vi "Front_measurement.vi"(8 "error in":errorcluster, 10 "AI duration (ms)":i32=1000, 11 "Digital Ports":tag="Dev1/port0") -> (1 "error out":errorcluster, 2 "data":waveform(dbl))   [LabVIEW 2021]
uses:
  <vilib>/DAQmx/write.llb/DAQmx Write (Digital 1D U32 1Chan NSamp).vi
  <vilib>/DAQmx/read.llb/DAQmx Read (Analog Wfm 1Chan NSamp).vi
  <vilib>/DAQmx/create/channels.llb/DAQmx Create Channel (DO-Digital Output).vi
  <vilib>/DAQmx/create/channels.llb/DAQmx Create Channel (CO-Pulse Generation-Ticks).vi
  <vilib>/DAQmx/configure/timing.llb/DAQmx Timing (Implicit).vi
  <vilib>/DAQmx/create/channels.llb/DAQmx Create Channel (AI-Voltage-Basic).vi
  <vilib>/DAQmx/configure/timing.llb/DAQmx Timing (Sample Clock).vi
  <vilib>/DAQmx/configure/trigger.llb/DAQmx Start Trigger (Analog Edge).vi
  Addons/DAQ_Pulse_Gen/Global_DAQ.vi
  <vilib>/DAQmx/miscellaneous.llb/DAQmx Fill In Error Info.vi
  <vilib>/DAQmx/create/channels.llb/DAQmx Create Channel (CO-Pulse Generation-Frequency).vi
  <vilib>/Utility/error.llb/Error Cluster From Error Code.vi
  <vilib>/ErrorRing/Error Ring.xnode
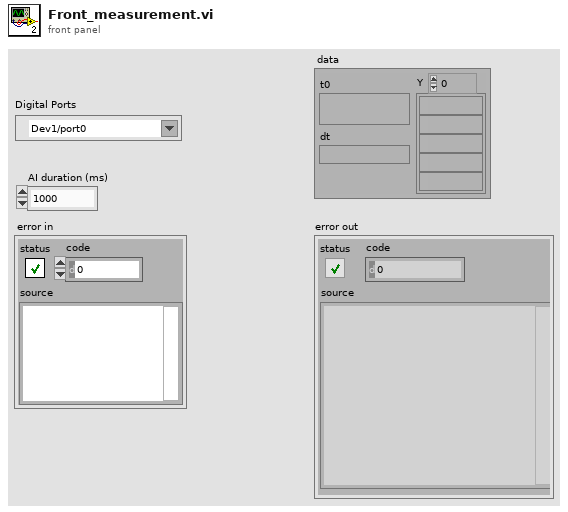
[diagram p1: front panel]
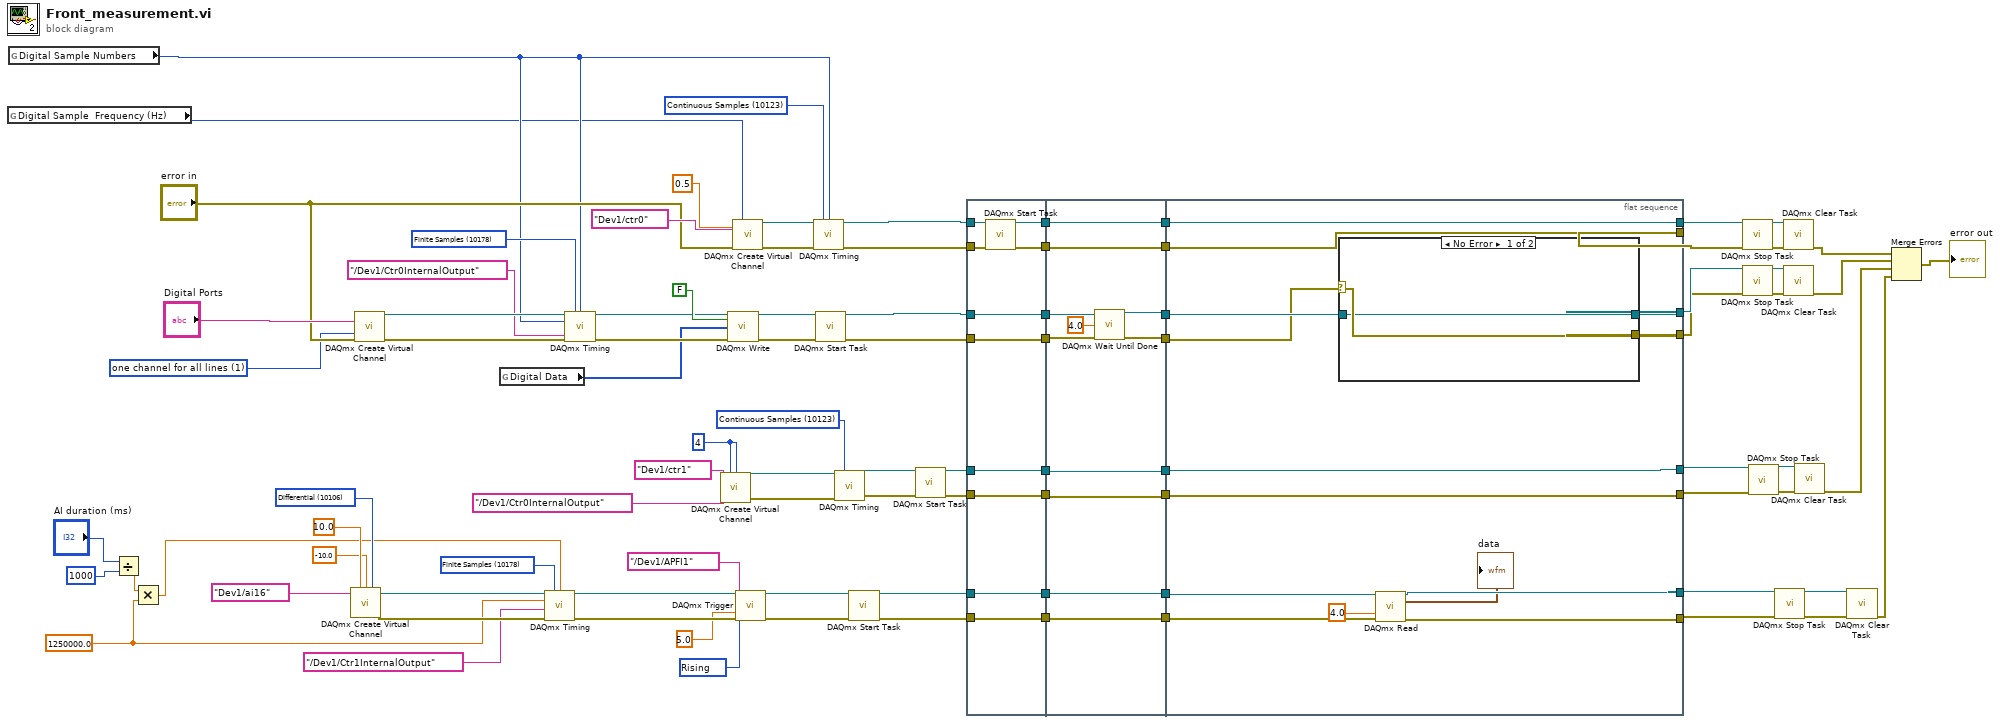
[diagram p0: block diagram]
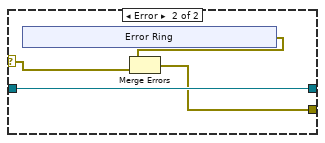
[diagram p2: hidden frame]
diagram:
  w3 = 1250000.0 ("rate")
  w26 = 10106 items=["Default"=-1, "RSE"=10083, "NRSE"=10078, "Differential"=10106, "Pseudodifferential"=12529] ("input terminal configuration")
  w28 = 10280 items=["Rising"=10280, "Falling"=10171] ("slope")
  w37 = 10178 items=["Finite Samples"=10178, "Continuous Samples"=10123, "Hardware Timed Single Point"=12522] ("sample mode")
  w55 = 10123 items=["Finite Samples"=10178, "Continuous Samples"=10123, "Hardware Timed Single Point"=12522] ("sample mode")
  w56 = u32 4 ("low ticks")
  w76 = 1 items=["one channel for each line", "one channel for all lines"] ("line grouping")
  w78 = 10123 items=["Finite Samples"=10178, "Continuous Samples"=10123, "Hardware Timed Single Point"=12522] ("sample mode")
  w86 = 10178 items=["Finite Samples"=10178, "Continuous Samples"=10123, "Hardware Timed Single Point"=12522] ("sample mode")
  n1 = global read "Global_DAQ.vi" "Digital Sample  Frequency (Hz)"() -> (w6:u32)
  n2 = global read "Global_DAQ.vi" "Digital Sample Numbers"() -> (w9:u32)
  n3 = Divide(x="AI duration (ms)", y=1000) -> (x/y=w4:dbl)
  n4 = Multiply(x=w4, y=w3) -> (x*y=w1:dbl)
  n5 = call-poly <vilib>:"DAQmx Create Virtual Channel.vi"("maximum value"=10.0, "minimum value"=-10.0, "input terminal configuration"=w26, "physical channels"=tag "Dev1/ai16") -> ("task out"=w47:refnum<k21>, "error out"=w46:errorcluster)  [unwired: 10 in]
  n6 = call-poly <vilib>:"DAQmx Create Virtual Channel.vi"("lines"="Digital Ports", "line grouping"=w76, "error in"="error in") -> ("task out"=w89:refnum<k21>, "error out"=w88:errorcluster)  [unwired: 11 in]
  n7 = global read "Global_DAQ.vi" "Digital Data"() -> (w77:u32[])
  n8 = call-poly <vilib>:"DAQmx Timing.vi"("task/channels in"=w47, "sample mode"=w37, "samples per channel"=w1, "rate"=w3, "source"=tag "/Dev1/Ctr1InternalOutput", "error in"=w46) -> ("task out"=w44:refnum<k21>, "error out"=w43:errorcluster)  [unwired: 8 in]
  n9 = call-poly <vilib>:"DAQmx Timing.vi"("task/channels in"=w89, "sample mode"=w86, "samples per channel"=w9, "rate"=w9, "source"=tag "/Dev1/Ctr0InternalOutput", "error in"=w88) -> ("task out"=w80:refnum<k21>, "error out"=w79:errorcluster)  [unwired: 8 in]
  n10 = call-poly <vilib>:"DAQmx Create Virtual Channel.vi"("high ticks"=w56, "low ticks"=w56, "counter"=tag "Dev1/ctr1", "source of ticks"=tag "/Dev1/Ctr0InternalOutput") -> ("task out"=w58:refnum<k21>, "error out"=w57:errorcluster)  [unwired: 10 in]
  n11 = call-poly <vilib>:"DAQmx Write.vi"("task/channels in"=w80, "auto start"=FALSE, "data"=w77, "error in"=w79) -> ("task out"=w83:refnum<k21>, "error out"=w82:errorcluster)  [unwired: 9 in, 1 out]
  n12 = call-poly <vilib>:"DAQmx Create Virtual Channel.vi"("frequency"=w6, "duty cycle"=0.5, "counter"=tag "Dev1/ctr0", "error in"="error in") -> ("task out"=w84:refnum<k21>, "error out"=w90:errorcluster)  [unwired: 10 in]
  n13 = call-poly <vilib>:"DAQmx Trigger.vi"("task/channels in"=w44, "source"=tag "/Dev1/APFI1", "slope"=w28, "level"=5.0, "error in"=w43) -> ("task out"=w41:refnum<k21>, "error out"=w40:errorcluster)  [unwired: 9 in]
  n14 = call-poly <vilib>:"DAQmx Timing.vi"("task/channels in"=w84, "sample mode"=w78, "samples per channel"=w9, "error in"=w90) -> ("task out"=w64:refnum<k21>, "error out"=w63:errorcluster)  [unwired: 10 in]
  n15 = call <vilib>:"DAQmx Start Task.vi"("task/channels in"=w83, "error in"=w82) -> ("task out"=w62:refnum<k21>, "error out"=w61:errorcluster)  [unwired: 12 in]
  n16 = call-poly <vilib>:"DAQmx Timing.vi"("task/channels in"=w58, "sample mode"=w55, "error in"=w57) -> ("task out"=w54:refnum<k21>, "error out"=w53:errorcluster)  [unwired: 11 in]
  n17 = call <vilib>:"DAQmx Start Task.vi"("task/channels in"=w41, "error in"=w40) -> ("task out"=w39:refnum<k21>, "error out"=w38:errorcluster)  [unwired: 12 in]
  n18 = call <vilib>:"DAQmx Start Task.vi"("task/channels in"=w54, "error in"=w53) -> ("task out"=w52:refnum<k21>, "error out"=w51:errorcluster)  [unwired: 12 in]
  n19 = flat-sequence {
    tunnel: [w101] -> w25
    tunnel: [w100] -> w23
    tunnel: [w99] -> w21
    tunnel: [w98] -> w19
    tunnel: w64 -> [w103]
    tunnel: w63 -> [w102]
    tunnel: w62 -> [w99]
    tunnel: w61 -> [w98]
    tunnel: w52 -> [w97]
    tunnel: w51 -> [w96]
    tunnel: w39 -> [w95]
    tunnel: w38 -> [w94]
    tunnel: [w97] -> w17
    tunnel: [w96] -> w15
    tunnel: [w95] -> w13
    tunnel: [w94] -> w11
    tunnel: w25 -> [w114]
    tunnel: [w114] -> w24
    tunnel: w23 -> [w113]
    tunnel: [w113] -> w22
    tunnel: w21 -> [w110]
    tunnel: [w108] -> w20
    tunnel: w19 -> [w109]
    tunnel: [w107] -> w18
    tunnel: w17 -> [w105]
    tunnel: [w105] -> w16
    tunnel: w15 -> [w104]
    tunnel: [w104] -> w14
    tunnel: w13 -> [w112]
    tunnel: [w112] -> w12
    tunnel: w11 -> [w111]
    tunnel: [w111] -> w10
    tunnel: w24 -> [w128]
    tunnel: w22 -> [w125]
    tunnel: w20 -> [w120]
    tunnel: w18 -> [w119]
    tunnel: [w128] -> w71
    tunnel: [w127] -> w68
    tunnel: [w126] -> w70
    tunnel: [w125] -> w69
    tunnel: w16 -> [w118]
    tunnel: w14 -> [w117]
    tunnel: w12 -> [w124]
    tunnel: w10 -> [w123]
    tunnel: [w118] -> w36
    tunnel: [w117] -> w35
    tunnel: [w122] -> w30
    tunnel: [w121] -> w29
    frame #0 {
      n20 = call <vilib>:"DAQmx Start Task.vi"("task/channels in"=w103, "error in"=w102) -> ("task out"=w101:refnum<k21>, "error out"=w100:errorcluster)  [unwired: 12 in]
    }
    frame #1 {
      n21 = call <vilib>:"DAQmx Wait Until Done.vi"("task/channels in"=w110, "timeout (sec)"=4.0, "error in"=w109) -> ("task out"=w108:refnum<k21>, "error out"=w107:errorcluster)  [unwired: 11 in]
    }
    frame #2 {
      n22 = case shown="No Error" w119 {
        selector: w119 -> [w130 w132]
        tunnel: [w130 w131] -> w127
        tunnel: w120 -> [w129 w134]
        tunnel: [w129 w134] -> w126
        frame No Error {
        }
        frame Error {
          n23 = xnode "Error Ring"() -> ("error out"=w133:errorcluster)
          n24 = Merge Errors(w133, w132) -> (w131:errorcluster)
        }
      }
      n25 = call-poly <vilib>:"DAQmx Read.vi"("task/channels in"=w124, "timeout"=4.0, "error in"=w123) -> ("task out"=w122:refnum<k21>, "data"=→"data":waveform(dbl), "error out"=w121:errorcluster)  [unwired: 10 in]
    }
  }
  n26 = call <vilib>:"DAQmx Stop Task.vi"("task/channels in"=w71, "error in"=w69) -> ("task out"=w73:refnum<k21>, "error out"=w72:errorcluster)  [unwired: 12 in]
  n27 = call <vilib>:"DAQmx Stop Task.vi"("task/channels in"=w70, "error in"=w68) -> ("task out"=w75:refnum<k21>, "error out"=w74:errorcluster)  [unwired: 12 in]
  n28 = call <vilib>:"DAQmx Stop Task.vi"("task/channels in"=w36, "error in"=w35) -> ("task out"=w34:refnum<k21>, "error out"=w33:errorcluster)  [unwired: 12 in]
  n29 = call <vilib>:"DAQmx Stop Task.vi"("task/channels in"=w30, "error in"=w29) -> ("task out"=w32:refnum<k21>, "error out"=w31:errorcluster)  [unwired: 12 in]
  n30 = call <vilib>:"DAQmx Clear Task.vi"("task in"=w73, "error in"=w72) -> ("error out"=w67:errorcluster)  [unwired: 13 in]
  n31 = call <vilib>:"DAQmx Clear Task.vi"("task in"=w75, "error in"=w74) -> ("error out"=w66:errorcluster)  [unwired: 13 in]
  n32 = call <vilib>:"DAQmx Clear Task.vi"("task in"=w34, "error in"=w33) -> ("error out"=w8:errorcluster)  [unwired: 13 in]
  n33 = call <vilib>:"DAQmx Clear Task.vi"("task in"=w32, "error in"=w31) -> ("error out"=w7:errorcluster)  [unwired: 13 in]
  n34 = Merge Errors(w67, w66, w8, w7) -> (→"error out":errorcluster)
